vi "TCP-IP.CMDSYS.vi"(7 "Cmd":enum16{"Read", "Write"}(ring), 8 "错误输入（无错误）":errorcluster, 9 "Value":u8[](array[numeric]), 10 "Register":T1(ring), 11 "连接ID输入":refnum<k5>) -> (0 "错误输出":errorcluster, 1 "OP_Status":i16, 2 "Data_Out":u8[](array[numeric]) format="%02x", 3 "ok?":bool)   [LabVIEW 2012, in "Lib_UEL.ATE.lvlib" / "Lib_IPVoice.lvlib"]
uses:
  Lib_IPVoice.lvlib
panel:
  out "无符号字节数组":u8[](array[numeric]) format="%02x"
  # "说明:\nOP_Status返回正数时,为数据长度\nOP_Status返回-1时,为对只读变量进行的写操作的错误代码.\n\n版本历史:\nV01."
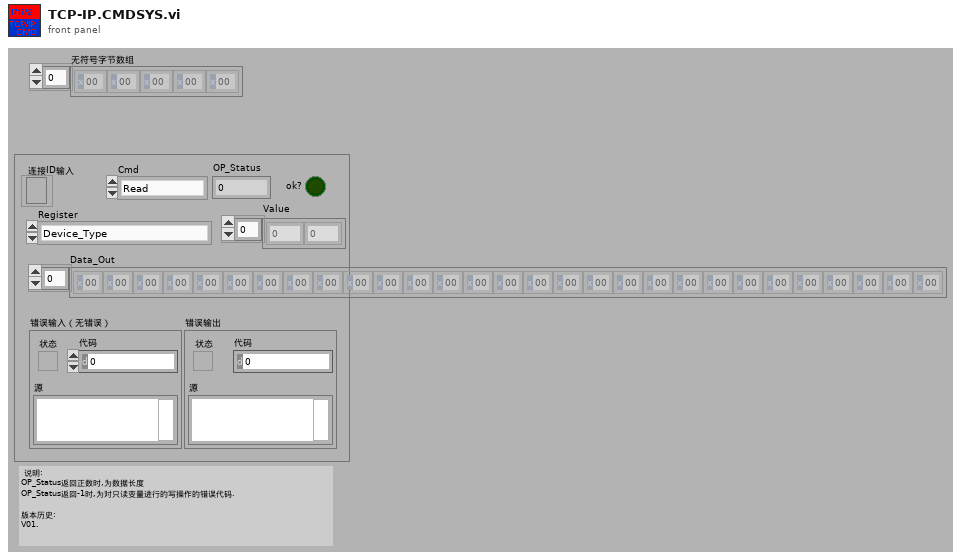
[diagram p1: front panel]
types:
  T1 = enum16{"Device_Type", "FWVersion", "debugmode", "sw_upgr_avail", "dbg_serial", "dbg_touch", "dbg_touch_x", "dbg_touch_y", "dbg_sd_status", "dbg_sd_write", "dbg_sd_write_res", "dbg_bright", "dbg_usb", "dbg_usb_res", "dbg_usb_sc", "dbg_ila", "dbg_hs", "dbg_hs_push", "dbg_hs_rec", "dbg_hs_rec_res", "dbg_hs_play", "dbg_led_mute", "dbg_led_allarm", "dbg_led_message", "dbg_led_door", "dbg_led_logo", "dbg_led_logo1", "dbg_aux_ring", "dbg_floor_call", "dbg_panic", "dbg_soft_on", "dbg_wifi", "dbg_wifi_res", "dbg_calibr_status", "dbg_calibr_status_res", "dbg_delta_cal", "dbg_calibrate", "dbg_calibrate_res", "dbg_audioin", "dbg_audioin_res", "dbg_audioin_offset", "dbg_audioout_left", "dbg_audioout_left_offset", "dbg_audioout_right", "dbg_audioout_right_offset", "dbg_audioout_6dB", "dbg_display", "dbg_video_loopback", "dbg_mac1", "dbg_mac2", "dbg_mac_wifi", "dbg_mac_bt", "dbg_mac_zigbee", "dbg_touch_aux", "dbg_audioout_mono", "dbg_touch_out"}
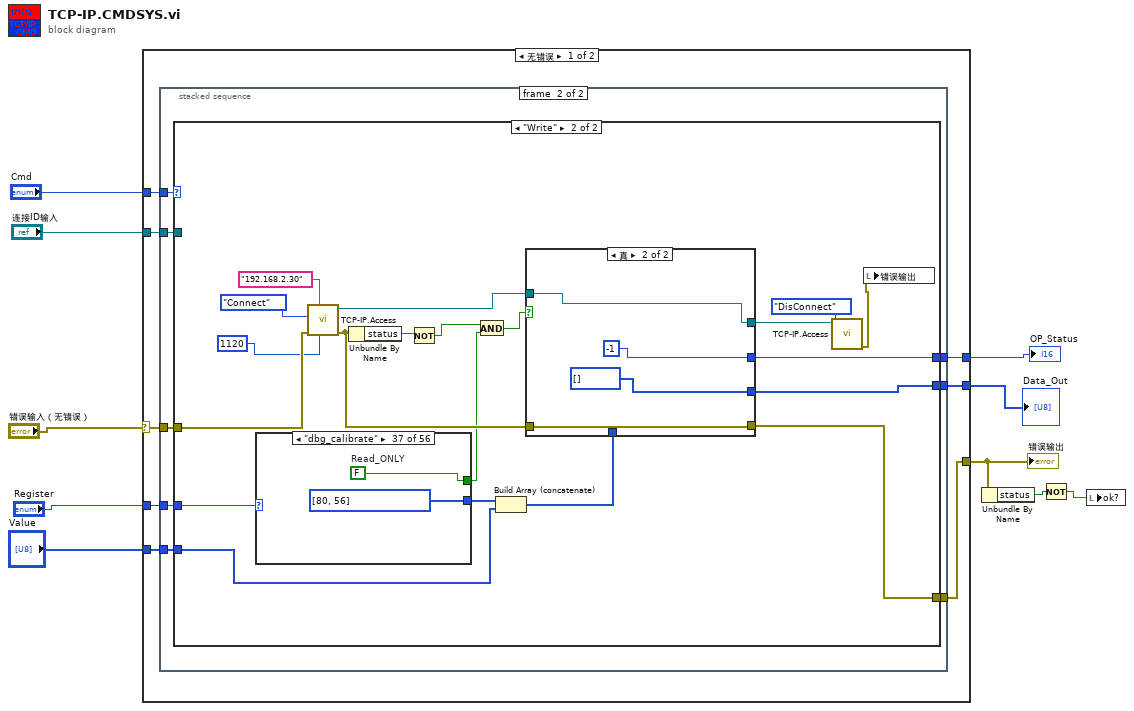
[diagram p0: block diagram]
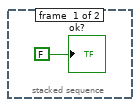
[diagram p2: hidden frame]
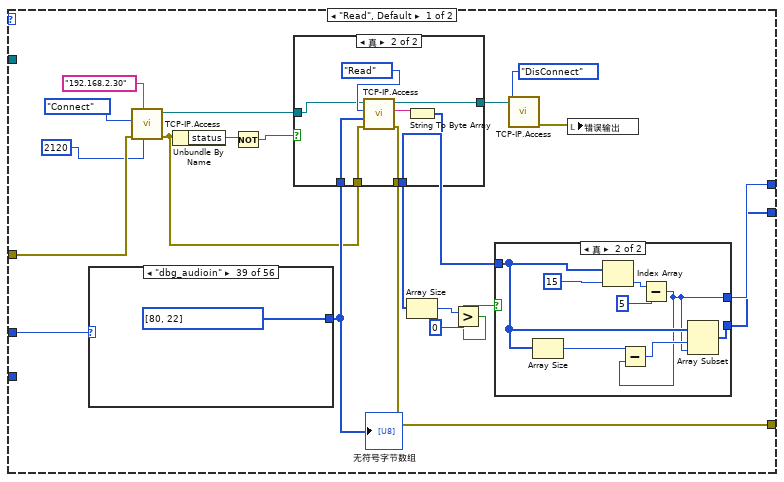
[diagram p3: hidden frame]
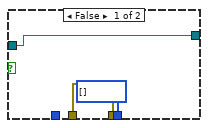
[diagram p4: hidden frame]
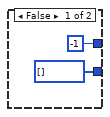
[diagram p5: hidden frame]
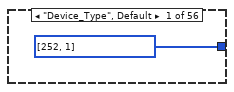
[diagram p6: hidden frame]
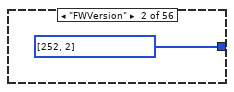
[diagram p7: hidden frame]
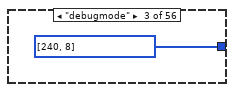
[diagram p8: hidden frame]
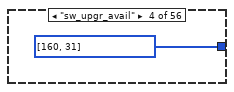
[diagram p9: hidden frame]
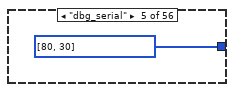
[diagram p10: hidden frame]
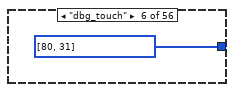
[diagram p11: hidden frame]
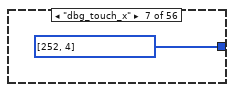
[diagram p12: hidden frame]
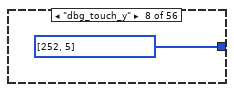
[diagram p13: hidden frame]
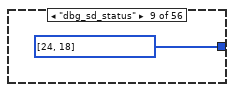
[diagram p14: hidden frame]
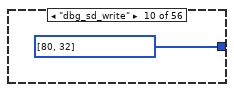
[diagram p15: hidden frame]
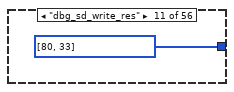
[diagram p16: hidden frame]
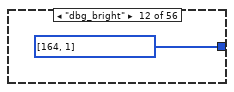
[diagram p17: hidden frame]
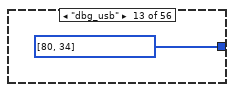
[diagram p18: hidden frame]
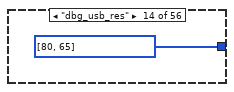
[diagram p19: hidden frame]
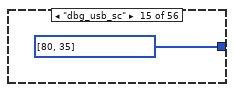
[diagram p20: hidden frame]
diagram:
  n1 = case shown="无错误" "错误输入（无错误）" {
    selector: "错误输入（无错误）" -> [w15 w272]
    tunnel: [w12 w272] -> w4
    tunnel: "Cmd" -> [w18 _]
    tunnel: "连接ID输入" -> [w17 _]
    tunnel: "Register" -> [w16 _]
    tunnel: [w14 -2] -> w6
    tunnel: [w13 u8[] [] ("unsigned byte array")] -> w5
    tunnel: "Value" -> [w11 _]
    frame No Error {
      n2 = stacked-sequence {
        tunnel: w18 -> [_ w27]
        tunnel: w17 -> [_ w26]
        tunnel: w16 -> [_ w25]
        tunnel: w15 -> [_ w24]
        tunnel: [_ w23] -> w14
        tunnel: [_ w22] -> w13
        tunnel: [_ w21] -> w12
        tunnel: w11 -> [_ w20]
        frame #0 {
          "ok?" <- FALSE ("ok?")
        }
        frame #1 {
          n3 = case shown="\"Write\"" w27 {
            tunnel: w26 -> [_ _]
            tunnel: w25 -> [w47 w144]
            tunnel: w24 -> [w38 w137]
            tunnel: [w44 w141] -> w23
            tunnel: [w43 w140] -> w22
            tunnel: [w46 w139] -> w21
            tunnel: w20 -> [_ w142]
            frame "Read", Default {
              n4 = case shown="\"dbg_audioin\"" w47 {
                tunnel: [u8[] [252, 1] ("无符号字节数组") u8[] [252, 2] ("无符号字节数组") u8[] [240, 8] ("无符号字节数组") u8[] [160, 31] ("无符号字节数组") u8[] [80, 30] ("无符号字节数组") u8[] [80, 31] ("无符号字节数组") u8[] [252, 4] ("无符号字节数组") u8[] [252, 5] ("无符号字节数组") u8[] [24, 18] ("无符号字节数组") u8[] [80, 32] ("无符号字节数组") u8[] [80, 33] ("无符号字节数组") u8[] [164, 1] ("无符号字节数组") u8[] [80, 34] ("无符号字节数组") u8[] [80, 65] ("无符号字节数组") u8[] [80, 35] ("无符号字节数组") u8[] [80, 36] ("无符号字节数组") u8[] [80, 37] ("无符号字节数组") u8[] [80, 38] ("无符号字节数组") u8[] [80, 39] ("无符号字节数组") u8[] [252, 6] ("无符号字节数组") u8[] [80, 41] ("无符号字节数组") u8[] [80, 42] ("无符号字节数组") u8[] [80, 43] ("无符号字节数组") u8[] [80, 44] ("无符号字节数组") u8[] [80, 45] ("无符号字节数组") u8[] [80, 46] ("无符号字节数组") u8[] [80, 47] ("无符号字节数组") u8[] [80, 48] ("无符号字节数组") u8[] [80, 49] ("无符号字节数组") u8[] [80, 50] ("无符号字节数组") u8[] [80, 51] ("无符号字节数组") u8[] [80, 52] ("无符号字节数组") u8[] [80, 53] ("无符号字节数组") u8[] [80, 54] ("无符号字节数组") u8[] [80, 55] ("无符号字节数组") u8[] [240, 243] ("无符号字节数组") u8[] [80, 56] ("无符号字节数组") u8[] [80, 57] ("无符号字节数组") u8[] [80, 22] ("无符号字节数组") u8[] [252, 7] ("无符号字节数组") u8[] [240, 241] ("无符号字节数组") u8[] [80, 23] ("无符号字节数组") u8[] [240, 240] ("无符号字节数组") u8[] [80, 24] ("无符号字节数组") u8[] [240, 242] ("无符号字节数组") u8[] [80, 66] ("无符号字节数组") u8[] [80, 64] ("无符号字节数组") u8[] [80, 29] ("无符号字节数组") u8[] [17, 16] ("无符号字节数组") u8[] [17, 17] ("无符号字节数组") u8[] [17, 18] ("无符号字节数组") u8[] [17, 19] ("无符号字节数组") u8[] [17, 20] ("无符号字节数组") u8[] [252, 8] ("无符号字节数组") u8[] [80, 58] ("无符号字节数组") u8[] [252, 8] ("无符号字节数组")] -> w45
                frame "Device_Type", Default {
                }
                frame "FWVersion" {
                }
                frame "debugmode" {
                }
                frame "sw_upgr_avail" {
                }
                frame "dbg_serial" {
                }
                frame "dbg_touch" {
                }
                frame "dbg_touch_x" {
                }
                frame "dbg_touch_y" {
                }
                frame "dbg_sd_status" {
                }
                frame "dbg_sd_write" {
                }
                frame "dbg_sd_write_res" {
                }
                frame "dbg_bright" {
                }
                frame "dbg_usb" {
                }
                frame "dbg_usb_res" {
                }
                frame "dbg_usb_sc" {
                }
                frame "dbg_ila" {
                }
                frame "dbg_hs" {
                }
                frame "dbg_hs_push" {
                }
                frame "dbg_hs_rec" {
                }
                frame "dbg_hs_rec_res" {
                }
                frame "dbg_hs_play" {
                }
                frame "dbg_led_mute" {
                }
                frame "dbg_led_allarm" {
                }
                frame "dbg_led_message" {
                }
                frame "dbg_led_door" {
                }
                frame "dbg_led_logo" {
                }
                frame "dbg_led_logo1" {
                }
                frame "dbg_aux_ring" {
                }
                frame "dbg_floor_call" {
                }
                frame "dbg_panic" {
                }
                frame "dbg_soft_on" {
                }
                frame "dbg_wifi" {
                }
                frame "dbg_wifi_res" {
                }
                frame "dbg_calibr_status" {
                }
                frame "dbg_calibr_status_res" {
                }
                frame "dbg_delta_cal" {
                }
                frame "dbg_calibrate" {
                }
                frame "dbg_calibrate_res" {
                }
                frame "dbg_audioin" {
                }
                frame "dbg_audioin_res" {
                }
                frame "dbg_audioin_offset" {
                }
                frame "dbg_audioout_left" {
                }
                frame "dbg_audioout_left_offset" {
                }
                frame "dbg_audioout_right" {
                }
                frame "dbg_audioout_right_offset" {
                }
                frame "dbg_audioout_6dB" {
                }
                frame "dbg_display" {
                }
                frame "dbg_video_loopback" {
                }
                frame "dbg_mac1" {
                }
                frame "dbg_mac2" {
                }
                frame "dbg_mac_wifi" {
                }
                frame "dbg_mac_bt" {
                }
                frame "dbg_mac_zigbee" {
                }
                frame "dbg_touch_aux" {
                }
                frame "dbg_audioout_mono" {
                }
                frame "dbg_touch_out" {
                }
              }
              "无符号字节数组" <- w45
              n5 = call "TCP-IP.Access.vi"("本地基端口"=u16 2120, "IP Address"="192.168.2.30", "错误输入（无错误）"=w38, "Command"=enum16{"Connect", "Read", "Write", "DisConnect"}."Connect") -> ("错误输出"=w37:errorcluster, "连接ID输出"=w36:refnum<k5>)  [unwired: 4 in, 2 out]
              n6 = Unbundle By Name(w37) -> ("status"=w30:bool)
              n7 = Not(x=w30) -> (.not. x?=w28:bool)
              n8 = case shown="真" w28 {
                tunnel: [w49 w56] -> w46
                tunnel: w45 -> [_ w55]
                tunnel: [u8[] [] ("unsigned byte array") w54] -> w42
                tunnel: w37 -> [w49 w53]
                tunnel: w36 -> [w50 w52]
                tunnel: [w50 w51] -> w35
                frame False {
                }
                frame True {
                  n9 = call "TCP-IP.Access.vi"("错误输入（无错误）"=w53, "CMD"=w55, "Command"=enum16{"Connect", "Read", "Write", "DisConnect"}."Read", "连接ID输入"=w52) -> ("错误输出"=w56:errorcluster, "数据输出"=w57:string, "连接ID输出"=w51:refnum<k5>)  [unwired: 4 in, 1 out]
                  n10 = String To Byte Array(string=w57) -> (unsigned byte array=w54:u8[])
                }
              }
              n11 = Array Size(array=w42) -> (size(s)=w41:i32)
              n12 = Greater?(x=w41, y=0) -> (0:w39:bool)
              n13 = case shown="真" w39 {
                tunnel: [i16 -1 w61] -> w44
                tunnel: [u8[] [] w63] -> w43
                tunnel: w42 -> [_ w62]
                frame False {
                }
                frame True {
                  n14 = Array Size(array=w62) -> (size(s)=w65:i32)
                  n15 = Index Array(array=w62, index=15 ("索引")) -> (element=w67:u8)
                  n16 = Subtract(x=w67, y=u8 5) -> (x-y=w61:u8)
                  n17 = Subtract(x=w65, y=w61) -> (x-y=w64:i32)
                  n18 = Array Subset(array=w62, index=w64, length=w61) -> (w63:u8[])
                }
              }
              n19 = call "TCP-IP.Access.vi"("Command"=enum16{"Connect", "Read", "Write", "DisConnect"}."DisConnect", "连接ID输入"=w35) -> ("错误输出"=w34:errorcluster)  [unwired: 6 in, 3 out]
              n20 = local write "错误输出"(w34) -> ()
            }
            frame "Write" {
              n21 = case shown="\"dbg_calibrate\"" w144 {
                tunnel: [u8[] [252, 1] ("无符号字节数组") u8[] [252, 2] ("无符号字节数组") u8[] [240, 8] ("无符号字节数组") u8[] [160, 31] ("无符号字节数组") u8[] [80, 30] ("无符号字节数组") u8[] [80, 31] ("无符号字节数组") u8[] [252, 4] ("无符号字节数组") u8[] [252, 5] ("无符号字节数组") u8[] [24, 18] ("无符号字节数组") u8[] [80, 32] ("无符号字节数组") u8[] [80, 33] ("无符号字节数组") u8[] [164, 1] ("无符号字节数组") u8[] [80, 34] ("无符号字节数组") u8[] [80, 65] ("无符号字节数组") u8[] [80, 35] ("无符号字节数组") u8[] [80, 36] ("无符号字节数组") u8[] [80, 37] ("无符号字节数组") u8[] [80, 38] ("无符号字节数组") u8[] [80, 39] ("无符号字节数组") u8[] [252, 6] ("无符号字节数组") u8[] [80, 41] ("无符号字节数组") u8[] [80, 42] ("无符号字节数组") u8[] [80, 43] ("无符号字节数组") u8[] [80, 44] ("无符号字节数组") u8[] [80, 45] ("无符号字节数组") u8[] [80, 46] ("无符号字节数组") u8[] [80, 47] ("无符号字节数组") u8[] [80, 48] ("无符号字节数组") u8[] [80, 49] ("无符号字节数组") u8[] [80, 50] ("无符号字节数组") u8[] [80, 51] ("无符号字节数组") u8[] [80, 52] ("无符号字节数组") u8[] [80, 53] ("无符号字节数组") u8[] [80, 54] ("无符号字节数组") u8[] [80, 55] ("无符号字节数组") u8[] [240, 243] ("无符号字节数组") u8[] [80, 56] ("无符号字节数组") u8[] [80, 57] ("无符号字节数组") u8[] [80, 22] ("无符号字节数组") u8[] [252, 7] ("无符号字节数组") u8[] [240, 241] ("无符号字节数组") u8[] [80, 23] ("无符号字节数组") u8[] [240, 240] ("无符号字节数组") u8[] [80, 24] ("无符号字节数组") u8[] [240, 242] ("无符号字节数组") u8[] [80, 66] ("无符号字节数组") u8[] [80, 64] ("无符号字节数组") u8[] [80, 29] ("无符号字节数组") u8[] [17, 16] ("无符号字节数组") u8[] [17, 17] ("无符号字节数组") u8[] [17, 18] ("无符号字节数组") u8[] [17, 19] ("无符号字节数组") u8[] [17, 20] ("无符号字节数组") u8[] [252, 8] ("无符号字节数组") u8[] [80, 58] ("无符号字节数组") u8[] [252, 8] ("无符号字节数组")] -> w143
                tunnel: [w158 w160 w162 w164 w166 w168 w170 w172 w174 w176 w178 w180 w182 w184 w186 w188 w190 w192 w194 w196 w198 w200 w202 w204 w206 w208 w210 w212 w214 w216 w218 w220 w222 w224 w226 w228 w230 w232 w234 w236 w238 w240 w242 w244 w246 w248 w250 w252 w254 w256 w258 w260 w262 w264 w266 w268] -> w126
                frame "Device_Type", Default {
                  w158 = TRUE  # Read_ONLY
                }
                frame "FWVersion" {
                  w160 = TRUE  # Read_ONLY
                }
                frame "debugmode" {
                  w162 = FALSE  # Read_ONLY
                }
                frame "sw_upgr_avail" {
                  w164 = FALSE  # Read_ONLY
                }
                frame "dbg_serial" {
                  w166 = FALSE  # Read_ONLY
                }
                frame "dbg_touch" {
                  w168 = FALSE  # Read_ONLY
                }
                frame "dbg_touch_x" {
                  w170 = TRUE  # Read_ONLY
                }
                frame "dbg_touch_y" {
                  w172 = TRUE  # Read_ONLY
                }
                frame "dbg_sd_status" {
                  w174 = TRUE  # Read_ONLY
                }
                frame "dbg_sd_write" {
                  w176 = FALSE  # Read_ONLY
                }
                frame "dbg_sd_write_res" {
                  w178 = TRUE  # Read_ONLY
                }
                frame "dbg_bright" {
                  w180 = FALSE  # Read_ONLY
                }
                frame "dbg_usb" {
                  w182 = TRUE  # Read_ONLY
                }
                frame "dbg_usb_res" {
                  w184 = TRUE  # Read_ONLY
                }
                frame "dbg_usb_sc" {
                  w186 = TRUE  # Read_ONLY
                }
                frame "dbg_ila" {
                  w188 = FALSE  # Read_ONLY
                }
                frame "dbg_hs" {
                  w190 = TRUE  # Read_ONLY
                }
                frame "dbg_hs_push" {
                  w192 = TRUE  # Read_ONLY
                }
                frame "dbg_hs_rec" {
                  w194 = FALSE  # Read_ONLY
                }
                frame "dbg_hs_rec_res" {
                  w196 = TRUE  # Read_ONLY
                }
                frame "dbg_hs_play" {
                  w198 = FALSE  # Read_ONLY
                }
                frame "dbg_led_mute" {
                  w200 = FALSE  # Read_ONLY
                }
                frame "dbg_led_allarm" {
                  w202 = FALSE  # Read_ONLY
                }
                frame "dbg_led_message" {
                  w204 = FALSE  # Read_ONLY
                }
                frame "dbg_led_door" {
                  w206 = FALSE  # Read_ONLY
                }
                frame "dbg_led_logo" {
                  w208 = FALSE  # Read_ONLY
                }
                frame "dbg_led_logo1" {
                  w210 = FALSE  # Read_ONLY
                }
                frame "dbg_aux_ring" {
                  w212 = FALSE  # Read_ONLY
                }
                frame "dbg_floor_call" {
                  w214 = TRUE  # Read_ONLY
                }
                frame "dbg_panic" {
                  w216 = TRUE  # Read_ONLY
                }
                frame "dbg_soft_on" {
                  w218 = TRUE  # Read_ONLY
                }
                frame "dbg_wifi" {
                  w220 = FALSE  # Read_ONLY
                }
                frame "dbg_wifi_res" {
                  w222 = TRUE  # Read_ONLY
                }
                frame "dbg_calibr_status" {
                  w224 = FALSE  # Read_ONLY
                }
                frame "dbg_calibr_status_res" {
                  w226 = TRUE  # Read_ONLY
                }
                frame "dbg_delta_cal" {
                  w228 = FALSE  # Read_ONLY
                }
                frame "dbg_calibrate" {
                  w230 = FALSE  # Read_ONLY
                }
                frame "dbg_calibrate_res" {
                  w232 = TRUE  # Read_ONLY
                }
                frame "dbg_audioin" {
                  w234 = FALSE  # Read_ONLY
                }
                frame "dbg_audioin_res" {
                  w236 = TRUE  # Read_ONLY
                }
                frame "dbg_audioin_offset" {
                  w238 = FALSE  # Read_ONLY
                }
                frame "dbg_audioout_left" {
                  w240 = FALSE  # Read_ONLY
                }
                frame "dbg_audioout_left_offset" {
                  w242 = FALSE  # Read_ONLY
                }
                frame "dbg_audioout_right" {
                  w244 = FALSE  # Read_ONLY
                }
                frame "dbg_audioout_right_offset" {
                  w246 = FALSE  # Read_ONLY
                }
                frame "dbg_audioout_6dB" {
                  w248 = FALSE  # Read_ONLY
                }
                frame "dbg_display" {
                  w250 = FALSE  # Read_ONLY
                }
                frame "dbg_video_loopback" {
                  w252 = FALSE  # Read_ONLY
                }
                frame "dbg_mac1" {
                  w254 = TRUE  # Read_ONLY
                }
                frame "dbg_mac2" {
                  w256 = TRUE  # Read_ONLY
                }
                frame "dbg_mac_wifi" {
                  w258 = TRUE  # Read_ONLY
                }
                frame "dbg_mac_bt" {
                  w260 = TRUE  # Read_ONLY
                }
                frame "dbg_mac_zigbee" {
                  w262 = TRUE  # Read_ONLY
                }
                frame "dbg_touch_aux" {
                  w264 = TRUE  # Read_ONLY
                }
                frame "dbg_audioout_mono" {
                  w266 = FALSE  # Read_ONLY
                }
                frame "dbg_touch_out" {
                  w268 = TRUE  # Read_ONLY
                }
              }
              n22 = call "TCP-IP.Access.vi"("本地基端口"=u16 1120, "IP Address"="192.168.2.30", "错误输入（无错误）"=w137, "Command"=enum16{"Connect", "Read", "Write", "DisConnect"}."Connect") -> ("错误输出"=w136:errorcluster, "连接ID输出"=w135:refnum<k5>)  [unwired: 4 in, 2 out]
              n23 = Unbundle By Name(w136) -> ("status"=w129:bool)
              n24 = Not(x=w129) -> (.not. x?=w127:bool)
              n25 = And(x=w127, y=w126) -> (x .and. y?=w125:bool)
              n26 = Build Array (concatenate)(w143, w142) -> (w138:u8[])
              n27 = case shown="真" w125 {
                tunnel: w135 -> [w153 w154]
                tunnel: [w147 -1] -> w141
                tunnel: [w148 u8[] [] ("unsigned byte array")] -> w140
                tunnel: [w150 w155] -> w139
                tunnel: w136 -> [w146 w155]
                tunnel: w138 -> [w151 _]
                tunnel: [w145 w154] -> w134
                frame False {
                  n28 = call "TCP-IP.Access.vi"("错误输入（无错误）"=w146, "CMD"=w151, "Command"=enum16{"Connect", "Read", "Write", "DisConnect"}."Write", "连接ID输入"=w153) -> ("错误输出"=w150:errorcluster, "数据输出"=w149:string, "连接ID输出"=w145:refnum<k5>)  [unwired: 4 in, 1 out]
                  n29 = String To Byte Array(string=w149) -> (unsigned byte array=w148:u8[])
                  n30 = Array Size(array=w148) -> (size(s)=w147:i32)
                }
                frame True {
                }
              }
              n31 = call "TCP-IP.Access.vi"("Command"=enum16{"Connect", "Read", "Write", "DisConnect"}."DisConnect", "连接ID输入"=w134) -> ("错误输出"=w133:errorcluster)  [unwired: 6 in, 3 out]
              n32 = local write "错误输出"(w133) -> ()
            }
          }
        }
      }
    }
    frame Error {
    }
  }
  "错误输出" <- w4
  "OP_Status" <- w6
  "Data_Out" <- w5
  n33 = Unbundle By Name(w4) -> ("status"=w3:bool)
  n34 = Not(x=w3) -> (.not. x?=w2:bool)
  n35 = local write "ok?"(w2) -> ()
